vi "lvDiff.vi"   [LabVIEW 2014]
uses:
  <vilib>/Utility/error.llb/DialogType.ctl
  <vilib>/lvrevbrd/DiffVIs.lvlib
  <vilib>/Wiresmith Technology/LabVIEW CLI/CLI Class/CLI.lvclass
types:
  T1 = typedef "DialogType.ctl" = u16
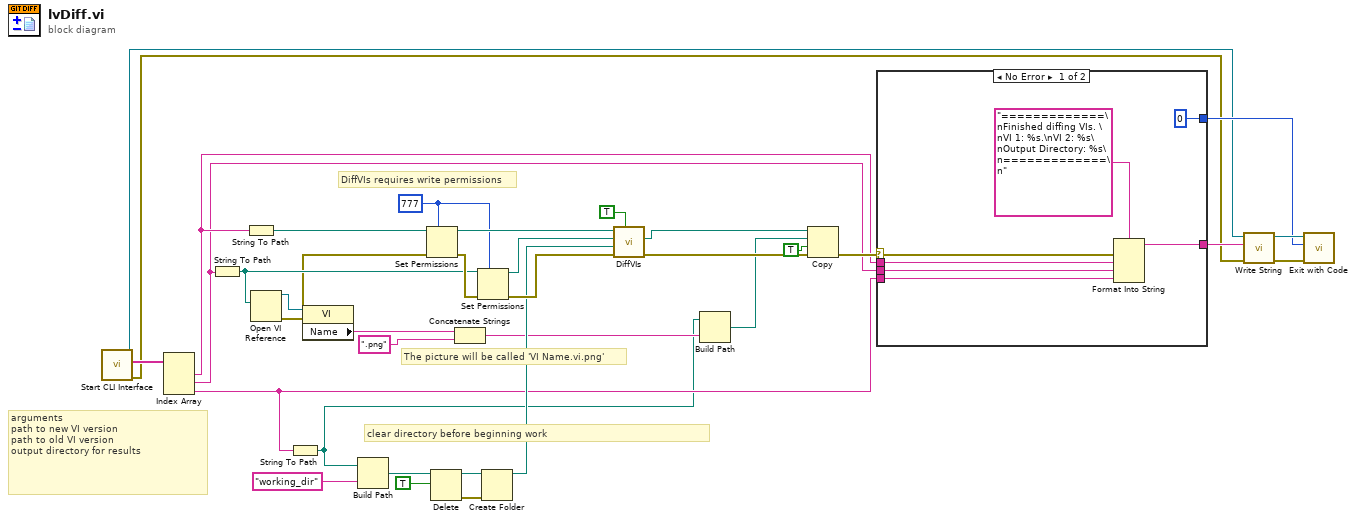
[diagram p0: block diagram]
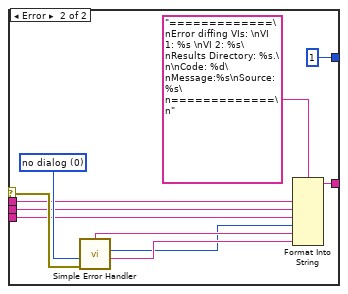
[diagram p2: hidden frame]
diagram:
  w13 = i16 777 ("permissions")
  # "clear directory before beginning work"
  # "DiffVIs requires write permissions"
  # "The picture will be called 'VI Name.vi.png'"
  # "arguments\npath to new VI version\npath to old VI version\noutput directory for results"
  n1 = call <vilib>:"Start CLI Interface.vi"() -> ("error out"=w11:errorcluster, "Custom Parameters"=w19:string[], "CLI out"=w20:refnum<class "CLI.lvclass">)  [unwired: 9 in]
  n2 = Index Array(array=w19) -> (element #1=w16:string, element #2=w14:string, element #3=w15:string)  [unwired: 3 in]
  n3 = String To Path(string=w14) -> (path=w9:path)
  n4 = String To Path(string=w16) -> (path=w29:path)
  n5 = Open VI Reference(vi path=w9) -> (vi reference=w8:refnum<vi>, error out=w7:errorcluster)  [unwired: 5 in]
  n6 = String To Path(string=w15) -> (path=w10:path)
  n7 = property class="VI"(reference=w8, error in=w7) -> (error out=w6:errorcluster, "Name"=w5:string)  [unwired: 1 out]
  n8 = Build Path(base path=w10, name or relative path="working_dir") -> (appended path=w3:path)
  n9 = Set Permissions(7:w13, 8:w6, 11:w29) -> (0:w18:errorcluster, 3:w34:path)  [unwired: 2 in]
  n10 = Delete(path (use dialog)=w3, entire hierarchy (F)=TRUE) -> (deleted path=w2:path, error out=w4:errorcluster)  [unwired: 3 in, 1 out]
  n11 = Concatenate Strings(w5, ".png" ("string")) -> (w27:string)
  n12 = Set Permissions(7:w13, 8:w18, 11:w9) -> (0:w35:errorcluster, 3:w33:path)  [unwired: 2 in]
  n13 = Create Folder(path (use dialog)=w2, error in=w4) -> (created path=w31:path)  [unwired: 1 in, 2 out]
  n14 = call <vilib>:"DiffVIs.vi"("Take ScrShots All In"=TRUE, "error in"=w35, "Picture Save Location"=w31, "VI Path 2"=w33, "VI Path 1"=w34) -> ("error out"=w30:errorcluster, "diff file"=w32:path)  [unwired: 2 in, 3 out]
  n15 = Build Path(base path=w10, name or relative path=w27) -> (appended path=w25:path)
  n16 = Copy(8:w30, 9:TRUE ("overwrite (F)"), 10:w25, 11:w32) -> (0:w17:errorcluster)  [unwired: 1 in, 2 out]
  n17 = case shown="No Error" w17 {
    selector: w17 -> [w42 w53]
    tunnel: [w41 w54] -> w24
    tunnel: [0 ("Exit Code (0)") 1 ("Exit Code (0)")] -> w22
    tunnel: w14 -> [w38 w45]
    tunnel: w15 -> [w37 w46]
    tunnel: w16 -> [w39 w44]
    frame No Error {
      n18 = Format Into String(format string="=============\nFinished diffing VIs. \nVI 1: %s.\nVI 2: %s\nOutput Directory: %s\n=============\n", error in=w42, w39, w38, w37) -> (resulting string=w41:string)  [unwired: 1 in, 1 out]
    }
    frame Error {
      w52 = T1 0 items=["no dialog", "OK message", "continue or stop message", "OK message + warnings", "continue/stop + warnings"] ("type of dialog (OK msg:1)")
      n19 = call <vilib>:"Simple Error Handler.vi"("type of dialog (OK msg:1)"=w52, "error in (no error)"=w53) -> ("code out"=w47:i32, "source out"=w48:string, "message"=w49:string)  [unwired: 3 in, 2 out]
      n20 = Format Into String(format string="=============\nError diffing VIs: \nVI 1: %s \nVI 2: %s\nResults Directory: %s.\n\nCode: %d\nMessage:%s\nSource: %s\n=============\n", w44, w45, w46, w47, w49, w48) -> (resulting string=w54:string)  [unwired: 2 in, 1 out]
    }
  }
  n21 = call <vilib>:"Write String.vi"("error in (no error)"=w11, "Text to Write"=w24, "CLI in"=w20) -> ("error out"=w21:errorcluster, "CLI out"=w23:refnum<class "CLI.lvclass">)  [unwired: 7 in]
  n22 = call <vilib>:"Exit with Code.vi"("error in (no error)"=w21, "Exit Code (0)"=w22, "CLI in"=w23) -> ()  [unwired: 8 in, 1 out]
